vi "Periodic Tasks.vi"(0 "error in":errorcluster) -> ()   [LabVIEW 2023]
doc: "All TeleOperated, Autonomous, and Test controller logic are located here. Sensor reads and actuator commands are run inside of parallel loops. Most FRC 4265 code should be placed here."
uses:
  GlobalMiscellaneous.vi
  GlobalDriverStationData.vi
  GlobalAutonomous.vi
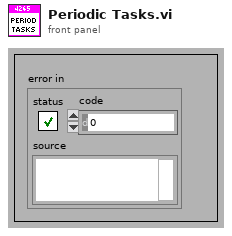
[diagram p1: front panel]
types:
  T1 = typedef "WPI_DriverStationRobotMode2.ctl" = enum16{"Autonomous Disabled", "Autonomous Enabled", "Teleop Disabled", "Teleop Enabled", "Disconnected", "Finish", "Test Disabled", "Test Enabled", "Emergency Stopped"}
  T2 = cluster{"Auto Error Out":errorcluster, "Drive Advance":bool, "Drive Step":i32, "Manipulator Step":i32, "Manipulator Advance":bool}
  T3 = cluster{"Auto Error":errorcluster, "Drive Advance":bool, "Drive Step":i32, "Manipulator Step":i32, "Manipulator Advance":bool}
  T4 = enum16{"Stow", "Speaker", "Amp", "Climbing", "Trap"}
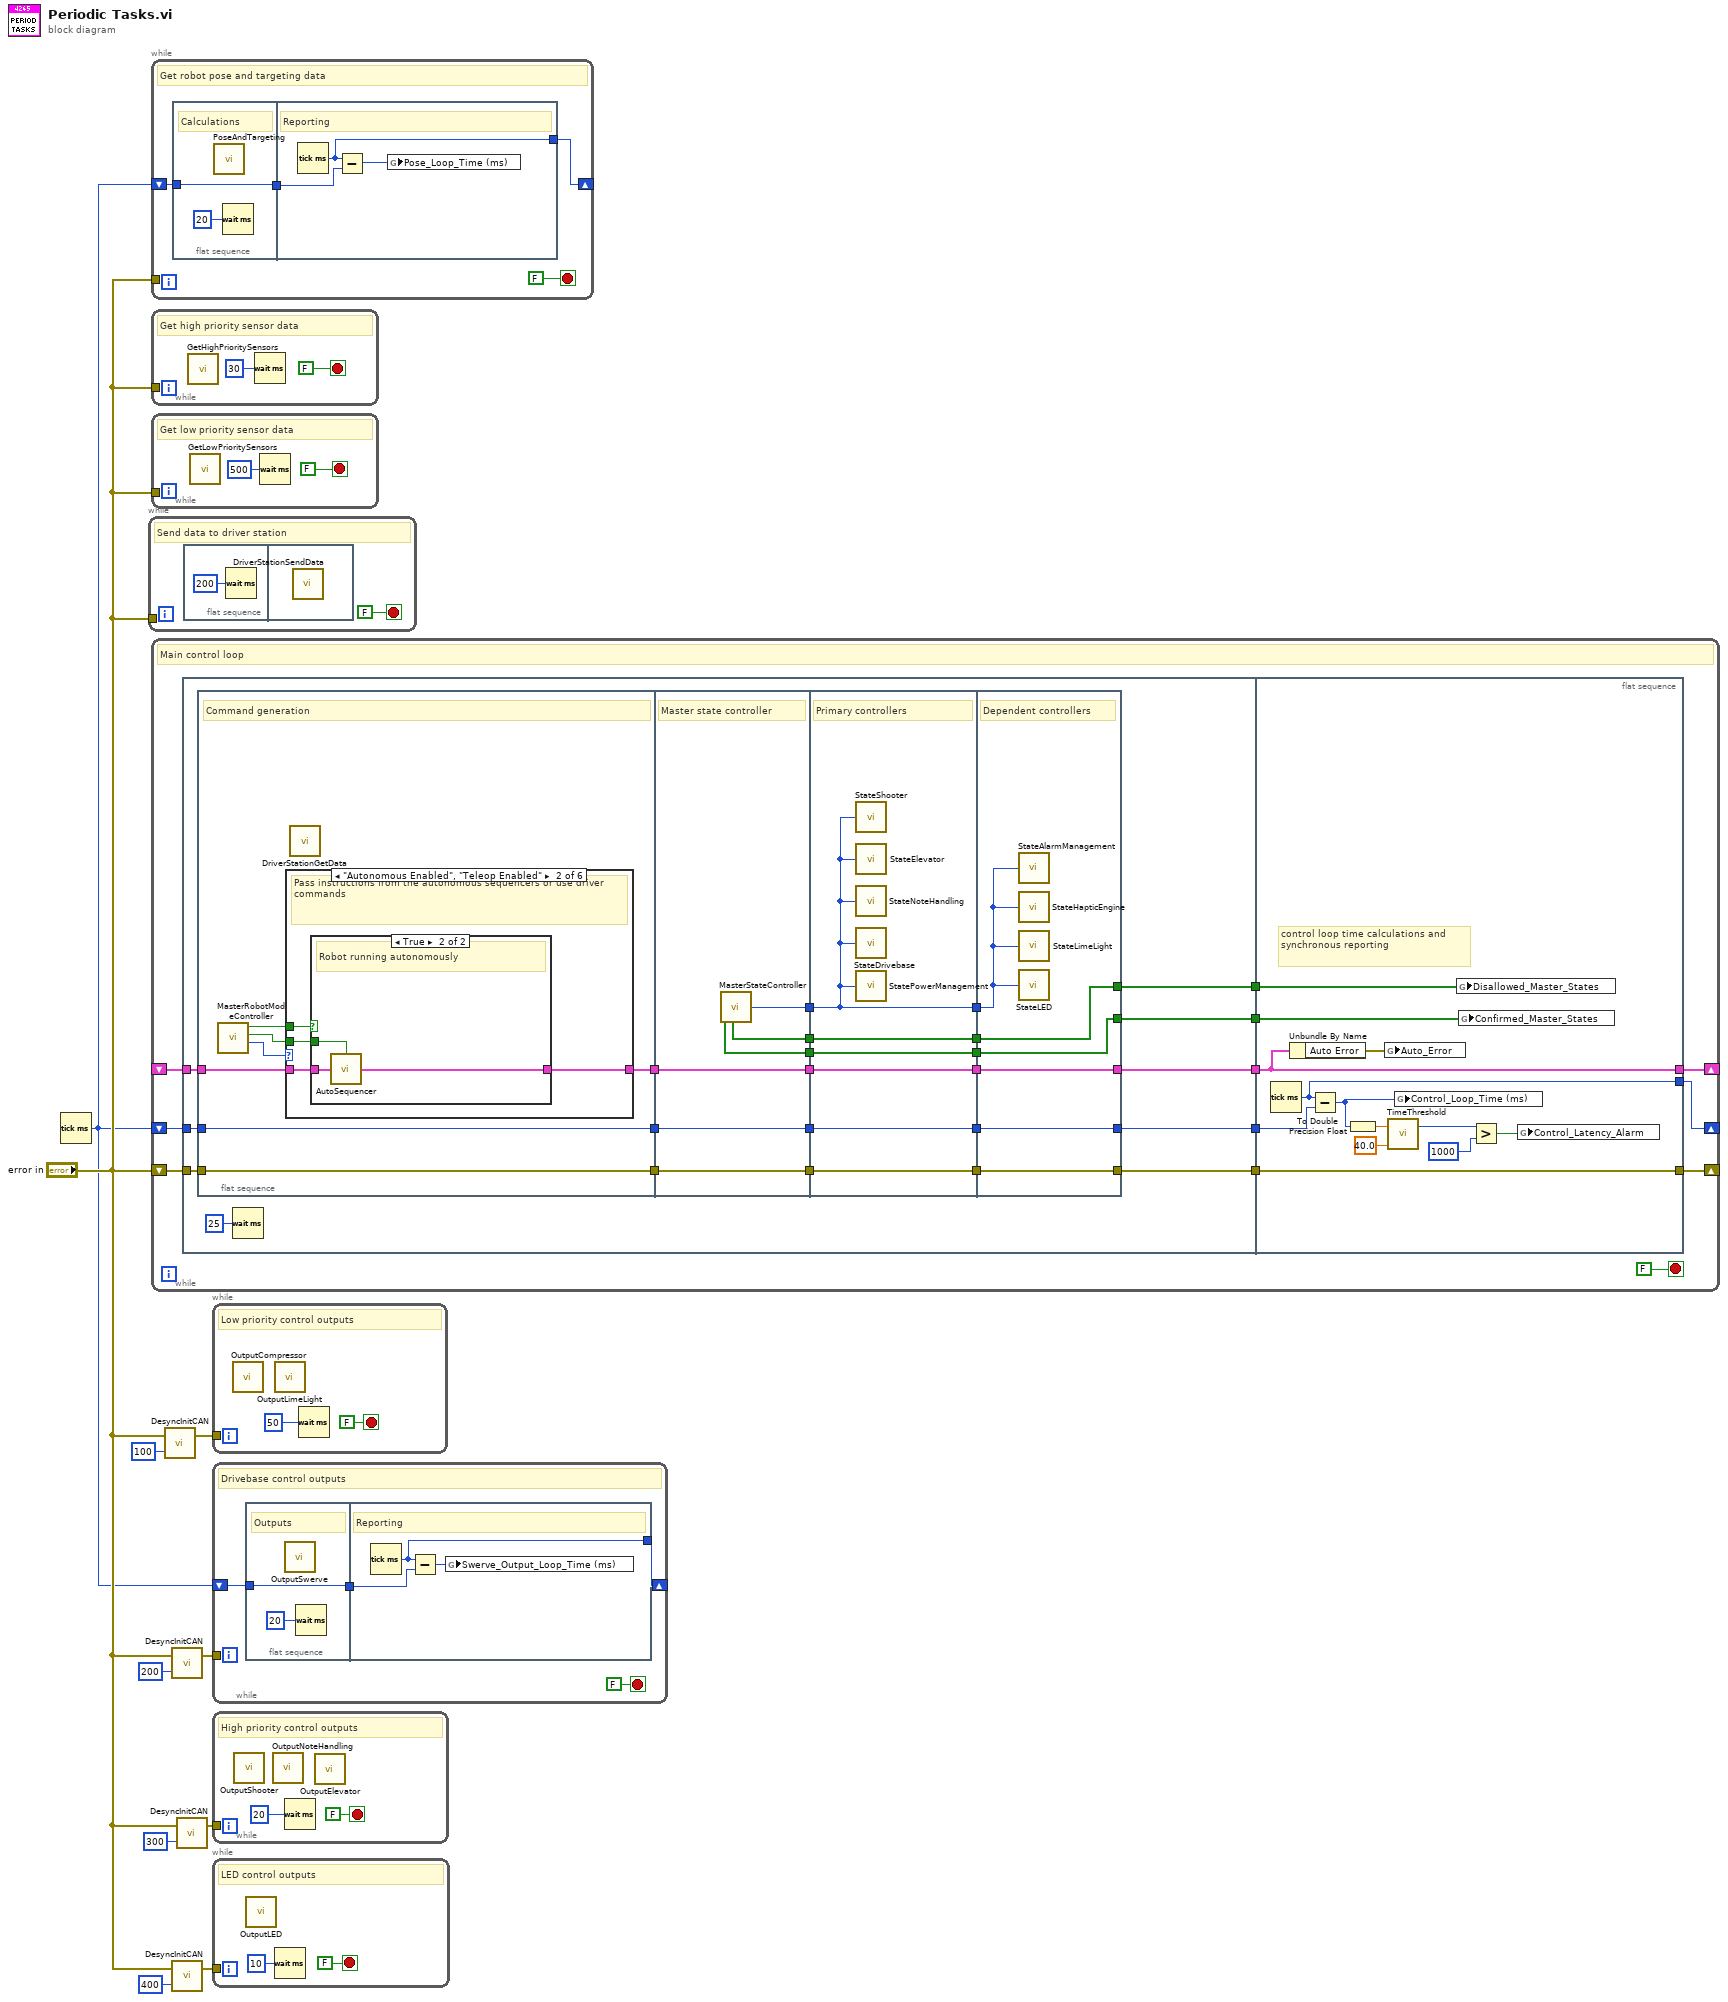
[diagram p0: block diagram]
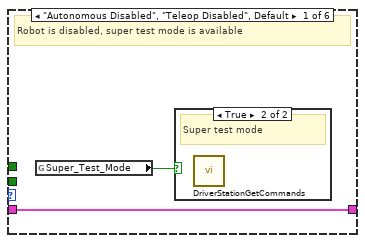
[diagram p2: hidden frame]
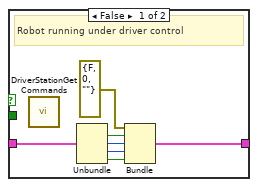
[diagram p4: hidden frame]
diagram:
  n1 = Tick Count (ms)() -> (millisecond timer value=w1:u32)
  n2 = while {
    tunnel: "error in" -> [_]
    stop <- FALSE stop-if-true
    # "Send data to driver station"
    n3 = flat-sequence {
      frame #0 {
        n4 = Wait (ms)(milliseconds to wait=u32 200) -> ()  [unwired: 1 out]
      }
      frame #1 {
        n5 = call "DriverStationSendData.vi"() -> ()  [unwired: 1 in]
      }
    }
  }
  n6 = while {
    tunnel: "error in" -> [_]
    shift-right: [w15] -> _
    shift-left: w1 -> [w14]
    stop <- FALSE stop-if-true
    # "Get robot pose and targeting data"
    n7 = flat-sequence {
      tunnel: w14 -> [w18]
      tunnel: [w18] -> w13
      tunnel: [w21] -> w15
      tunnel: w13 -> [w20]
      frame #0 {
        # "Calculations"
        n8 = call "PoseAndTargeting.vi"() -> ()  [unwired: 1 in]
        n9 = Wait (ms)(milliseconds to wait=u32 20) -> ()  [unwired: 1 out]
      }
      frame #1 {
        # "Reporting"
        n10 = Tick Count (ms)() -> (millisecond timer value=w21:u32)
        n11 = Subtract(x=w21, y=w20) -> (x-y=w19:u32)
        n12 = global write "GlobalMiscellaneous.vi" "Pose_Loop_Time (ms)"(w19) -> ()
      }
    }
  }
  n13 = while {
    tunnel: "error in" -> [_]
    stop <- FALSE stop-if-true
    # "Get high priority sensor data"
    n14 = call "GetHighPrioritySensors.vi"() -> ()  [unwired: 1 in]
    n15 = Wait (ms)(milliseconds to wait=u32 30) -> ()  [unwired: 1 out]
  }
  n16 = while {
    tunnel: "error in" -> [_]
    stop <- FALSE stop-if-true
    # "Get low priority sensor data"
    n17 = call "GetLowPrioritySensors.vi"() -> ()  [unwired: 1 in]
    n18 = Wait (ms)(milliseconds to wait=u32 500) -> ()  [unwired: 1 out]
  }
  n19 = while {
    shift-right: [w31] -> _
    shift-left: w1 -> [w32]
    shift-right: [w36] -> _
    shift-left: _ -> [w35]
    shift-right: [w33] -> _
    shift-left: "error in" -> [w34]
    stop <- FALSE stop-if-true
    # "Main control loop"
    n20 = flat-sequence {
      tunnel: w35 -> [w54]
      tunnel: w34 -> [w53]
      tunnel: w32 -> [w51]
      tunnel: [w55] -> w30
      tunnel: [w52] -> w29
      tunnel: [w49] -> w28
      tunnel: [w43] -> w27
      tunnel: [w40] -> w26
      tunnel: [w113] -> w31
      tunnel: [w119] -> w33
      tunnel: [w112] -> w36
      tunnel: w30 -> [w112]
      tunnel: w29 -> [w119]
      tunnel: w28 -> [w114]
      tunnel: w27 -> [w108]
      tunnel: w26 -> [w107]
      frame #0 {
        n21 = flat-sequence {
          tunnel: [w68] -> w61
          tunnel: w54 -> [w67]
          tunnel: [w63] -> w60
          tunnel: w53 -> [w63]
          tunnel: [w62] -> w59
          tunnel: w51 -> [w62]
          tunnel: [w94] -> w47
          tunnel: [w93] -> w46
          tunnel: w61 -> [w93]
          tunnel: w60 -> [w92]
          tunnel: [w92] -> w45
          tunnel: w59 -> [w91]
          tunnel: [w91] -> w44
          tunnel: [w90] -> w41
          tunnel: [w89] -> w38
          tunnel: w47 -> [w97]
          tunnel: [w100] -> w58
          tunnel: w46 -> [w100]
          tunnel: [w99] -> w57
          tunnel: w45 -> [w99]
          tunnel: [w98] -> w56
          tunnel: w44 -> [w98]
          tunnel: [w97] -> w48
          tunnel: [w96] -> w42
          tunnel: w41 -> [w96]
          tunnel: [w95] -> w39
          tunnel: w38 -> [w95]
          tunnel: [w106] -> w55
          tunnel: w58 -> [w106]
          tunnel: [w105] -> w52
          tunnel: w57 -> [w105]
          tunnel: w56 -> [w104]
          tunnel: [w104] -> w49
          tunnel: w48 -> [w103]
          tunnel: [w102] -> w43
          tunnel: w42 -> [w102]
          tunnel: [w101] -> w40
          tunnel: w39 -> [w101]
          frame #0 {
            # "Command generation"
            n22 = call "MasterRobotModeController.vi"() -> ("FMS Robot Mode"=w66:T1, "Auto Reset"=w65:bool, "Robot is Autonomous"=w64:bool)  [unwired: 5 in]
            n23 = case shown="\"Autonomous Enabled\", \"Teleop Enabled\"" w66 {
              tunnel: w65 -> [_ w72 _ _ _ _]
              tunnel: [w69 w74 w85 w86 w87 w88] -> w68
              tunnel: w67 -> [w69 w73 w85 w86 w87 w88]
              tunnel: w64 -> [_ w71 _ _ _ _]
              frame "Autonomous Disabled", "Teleop Disabled", Default {
                # "Robot is disabled, super test mode is available"
                n24 = global read "GlobalDriverStationData.vi" "Super_Test_Mode"() -> (w70:bool)
                n25 = case shown="True" w70 {
                  frame False {
                    # "Fully disabled"
                  }
                  frame True {
                    # "Super test mode"
                    n26 = call "DriverStationGetCommands.vi"() -> ()  [unwired: 12 in]
                  }
                }
              }
              frame "Autonomous Enabled", "Teleop Enabled" {
                # "Pass instructions from the autonomous sequencers or use driver commands"
                n27 = case shown="True" w71 {
                  tunnel: w72 -> [_ w84]
                  tunnel: [w80 w83] -> w74
                  tunnel: w73 -> [w81 w82]
                  frame False {
                    # "Robot running under driver control"
                    n28 = call "DriverStationGetCommands.vi"() -> ()  [unwired: 12 in]
                    n29 = Unbundle(w81) -> ("Drive Advance"=w76:bool, "Drive Step"=w77:i32, "Manipulator Step"=w78:i32, "Manipulator Advance"=w79:bool)  [unwired: 1 out]
                    n30 = Bundle("Auto Error Out"=errorcluster {"status"=FALSE, "code"=0, "source"=""}, "Drive Advance"=w76, "Drive Step"=w77, "Manipulator Step"=w78, "Manipulator Advance"=w79) -> (w80:T2)  [unwired: 1 in]
                  }
                  frame True {
                    # "Robot running autonomously"
                    n31 = call "AutoSequencer.vi"("Reinit Sequencer"=w84, "Auto Cluster In"=w82) -> ("Auto Cluster Out"=w83:T3)  [unwired: 13 in]
                  }
                }
              }
              frame "Finish" {
                # "Clean up operations are in the Finish.vi in RobotMain.vi"
              }
              frame "Test Disabled", "Test Enabled" {
                # "Use TestActuatorInterlock.vi for implimenting test code"
              }
              frame "Disconnected" {
                # "Communications have failed"
              }
              frame "Emergency Stopped" {
                # "Robot has been emergency stopped"
              }
            }
            n32 = call "DriverStationGetData.vi"() -> ()  [unwired: 1 in]
          }
          frame #1 {
            # "Master state controller"
            n33 = call "MasterStateController.vi"() -> ("Confirmed States"=w89:bool[], "Disallowed States"=w90:bool[], "Master State Out"=w94:T4)  [unwired: 3 in]
          }
          frame #2 {
            # "Primary controllers"
            n34 = call "StateShooter.vi"("Master State In"=w97) -> ()
            n35 = call "StateElevator.vi"("Master State In"=w97) -> ()
            n36 = call "StateNoteHandling.vi"("Master State In"=w97) -> ()
            n37 = call "StateDrivebase.vi"("Master State In"=w97) -> ()
            n38 = call "StatePowerManagement.vi"("Master State In"=w97) -> ()
          }
          frame #3 {
            # "Dependent controllers"
            n39 = call "StateAlarmManagement.vi"("Master State In"=w103) -> ()
            n40 = call "StateHapticEngine.vi"("Master State In"=w103) -> ()
            n41 = call "StateLimeLight.vi"("Master State In"=w103) -> ()
            n42 = call "StateLED.vi"("Master State In"=w103) -> ()
          }
        }
        n43 = Wait (ms)(milliseconds to wait=u32 25) -> ()  [unwired: 1 out]
      }
      frame #1 {
        # "control loop time calculations and synchronous reporting"
        n44 = Tick Count (ms)() -> (millisecond timer value=w113:u32)
        n45 = Unbundle By Name(w112) -> ("Auto Error"=w111:errorcluster)
        n46 = Subtract(x=w113, y=w114) -> (x-y=w110:u32)
        n47 = To Double Precision Float(number=w110) -> (double precision float=w118:dbl)
        n48 = global write "GlobalAutonomous.vi" "Auto_Error"(w111) -> ()
        n49 = call "TimeThreshold.vi"("Threshold"=40.0, "Current Value"=w118) -> ("Time Above Threshold (ms)"=w117:u32)  [unwired: 1 out]
        n50 = global write "GlobalMiscellaneous.vi" "Control_Loop_Time (ms)"(w110) -> ()
        n51 = global write "GlobalMiscellaneous.vi" "Disallowed_Master_States"(w108) -> ()
        n52 = global write "GlobalMiscellaneous.vi" "Confirmed_Master_States"(w107) -> ()
        n53 = Greater?(x=w117, y=u32 1000) -> (0:w109:bool)
        n54 = global write "GlobalMiscellaneous.vi" "Control_Latency_Alarm"(w109) -> ()
      }
    }
  }
  n55 = call "DesyncInitCAN.vi"("Desync Time (ms)"=u32 100, "error in"="error in") -> ("error out"=w10:errorcluster)  [unwired: 1 in]
  n56 = call "DesyncInitCAN.vi"("Desync Time (ms)"=u32 200, "error in"="error in") -> ("error out"=w7:errorcluster)  [unwired: 1 in]
  n57 = call "DesyncInitCAN.vi"("Desync Time (ms)"=u32 400, "error in"="error in") -> ("error out"=w3:errorcluster)  [unwired: 1 in]
  n58 = call "DesyncInitCAN.vi"("Desync Time (ms)"=u32 300, "error in"="error in") -> ("error out"=w5:errorcluster)  [unwired: 1 in]
  n59 = while {
    tunnel: w10 -> [_]
    stop <- FALSE stop-if-true
    # "Low priority control outputs"
    n60 = call "OutputCompressor.vi"() -> ()  [unwired: 1 in]
    n61 = call "OutputLimeLight.vi"() -> ()  [unwired: 1 in]
    n62 = Wait (ms)(milliseconds to wait=u32 50) -> ()  [unwired: 1 out]
  }
  n63 = while {
    tunnel: w7 -> [_]
    shift-right: [w122] -> _
    shift-left: w1 -> [w123]
    stop <- FALSE stop-if-true
    # "Drivebase control outputs"
    n64 = flat-sequence {
      tunnel: w123 -> [w127]
      tunnel: [w127] -> w124
      tunnel: [w130] -> w122
      tunnel: w124 -> [w129]
      frame #0 {
        # "Outputs"
        n65 = call "OutputSwerve.vi"() -> ()  [unwired: 1 in]
        n66 = Wait (ms)(milliseconds to wait=u32 20) -> ()  [unwired: 1 out]
      }
      frame #1 {
        # "Reporting"
        n67 = Tick Count (ms)() -> (millisecond timer value=w130:u32)
        n68 = Subtract(x=w130, y=w129) -> (x-y=w128:u32)
        n69 = global write "GlobalMiscellaneous.vi" "Swerve_Output_Loop_Time (ms)"(w128) -> ()
      }
    }
  }
  n70 = while {
    tunnel: w5 -> [_]
    stop <- FALSE stop-if-true
    # "High priority control outputs"
    n71 = call "OutputShooter.vi"() -> ()  [unwired: 1 in]
    n72 = call "OutputNoteHandling.vi"() -> ()  [unwired: 1 in]
    n73 = Wait (ms)(milliseconds to wait=u32 20) -> ()  [unwired: 1 out]
    n74 = call "OutputElevator.vi"() -> ()  [unwired: 1 in]
  }
  n75 = while {
    tunnel: w3 -> [_]
    stop <- FALSE stop-if-true
    # "LED control outputs"
    n76 = call "OutputLED.vi"() -> ()  [unwired: 1 in]
    n77 = Wait (ms)(milliseconds to wait=u32 10) -> ()  [unwired: 1 out]
  }
